vi "Error Handler.vi"(8 "error in":errorcluster) -> (0 "error out":errorcluster)   [LabVIEW 2021]
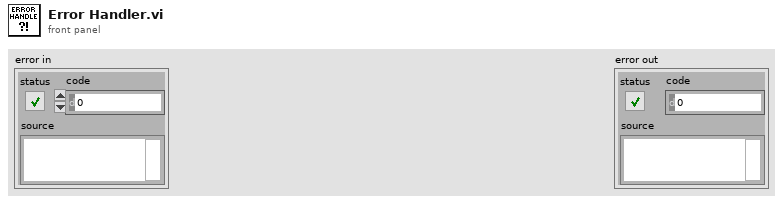
[diagram p1: front panel]
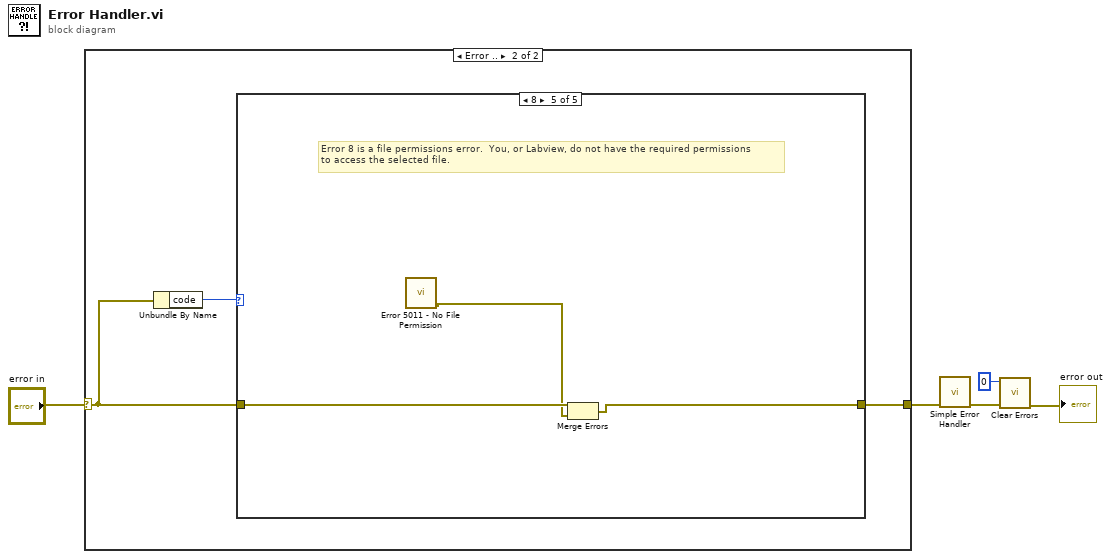
[diagram p0: block diagram]
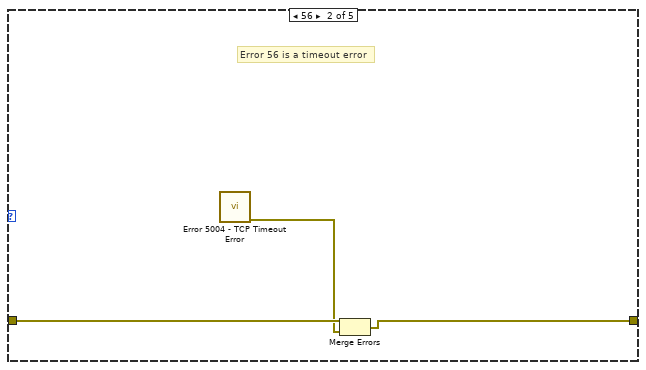
[diagram p4: hidden frame]
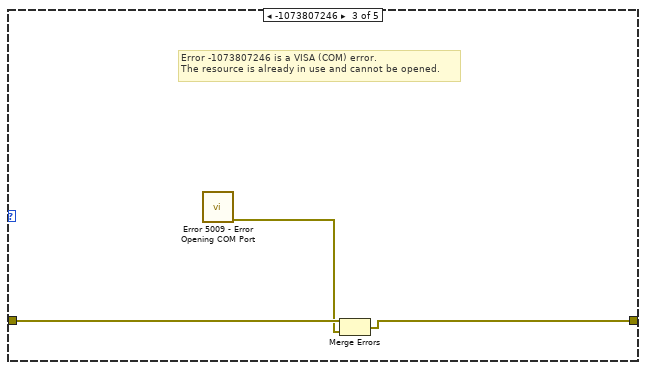
[diagram p5: hidden frame]
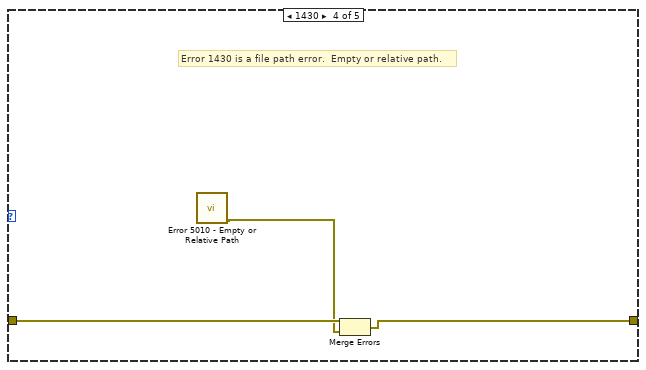
[diagram p6: hidden frame]
diagram:
  n1 = case shown="Error .." "error in" {
    selector: "error in" -> [w6 w8]
    tunnel: [w6 w7] -> w4
    frame No Error {
      # "No errors to handle"
    }
    frame Error {
      n2 = Unbundle By Name(w8) -> ("code"=w9:i32)
      n3 = case shown="8" w9 {
        tunnel: w8 -> [w10 w13 w16 w19 w22]
        tunnel: [w10 w11 w15 w18 w21] -> w7
        frame 0, Default {
          # "No error code, but error status is set to true"
        }
        frame 56 {
          # "Error 56 is a timeout error"
          n4 = call "Error 5004 - TCP Timeout Error.vi"() -> ("error out"=w12:errorcluster)  [unwired: 11 in]
          n5 = Merge Errors(w13, w12) -> (w11:errorcluster)
        }
        frame -1073807246 {
          # "Error -1073807246 is a VISA (COM) error.\nThe resource is already in use and cannot be opened."
          n6 = call "Error 5009 - Error Opening COM Port.vi"() -> ("error out"=w14:errorcluster)  [unwired: 11 in]
          n7 = Merge Errors(w16, w14) -> (w15:errorcluster)
        }
        frame 1430 {
          # "Error 1430 is a file path error.  Empty or relative path."
          n8 = call "Error 5010 - Empty or Relative Path.vi"() -> ("error out"=w17:errorcluster)  [unwired: 11 in]
          n9 = Merge Errors(w19, w17) -> (w18:errorcluster)
        }
        frame 8 {
          # "Error 8 is a file permissions error.  You, or Labview, do not have the required permissions\nto access the selected file."
          n10 = call "Error 5011 - No File Permission.vi"() -> ("error out"=w20:errorcluster)  [unwired: 11 in]
          n11 = Merge Errors(w22, w20) -> (w21:errorcluster)
        }
      }
    }
  }
  n12 = call <vilib>:"Simple Error Handler.vi"("error in (no error)"=w4) -> ("error out"=w3:errorcluster)  [unwired: 4 in, 4 out]
  n13 = call <vilib>:"Clear Errors.vi"("error in (no error)"=w3, "specific error code to clear (0: all)"=0) -> ("error out"=→"error out":errorcluster)  [unwired: 4 in, 1 out]
